vi "03-MonitorTemperatura.vi"() -> ()   [LabVIEW 2014]
panel:
  in  "Temp Scale":bool
  out "Temp historico":dbl(graph)
  in  "Power":bool
  # "ON"
  # "OFF"
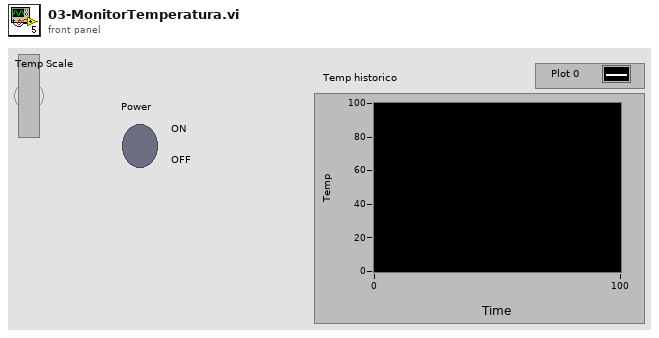
[diagram p1: front panel]
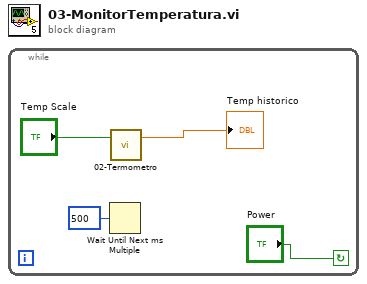
[diagram p0: block diagram]
diagram:
  n1 = while {
    stop <- "Power" continue-if-true
    n2 = Wait Until Next ms Multiple(millisecond multiple=u32 500) -> ()  [unwired: 1 out]
    n3 = call "02-Termometro.vi"("Temp Scale"="Temp Scale") -> ("Thermometer"=→"Temp historico":dbl)  [unwired: 2 in]
  }
